vi "SIRRectHole.vi"(8 "P":cluster{"x":dbl, "y":dbl, "z":dbl}={"x"=1.0, "y"=-5.0, "z"=1.0} {"x" format="%.2f"; "z" format="%.2f"; "y" format="%.2f"}, 9 "Variables":T1={"sound spd (cm/s)"=150000, "time step (s)"=1e-09} {"time step (s)" format="%.2e"}, 11 "strip":cluster{"Radius":dbl, "h":dbl, "a":dbl}={"Radius"=10.0, "h"=3.0, "a"=5.0} {"Radius" format="%.2f"; "a" format="%.2f"; "h" format="%.2f"}) -> (1 "lower":dbl[](graph), 2 "upper":dbl[](graph), 3 "h rect":dbl[](graph), 4 "delay out":i32, 5 "h cap":dbl[](array[numeric]) format="%.2f", 7 "cap delay pts":i32)   [LabVIEW 2022 SP3]
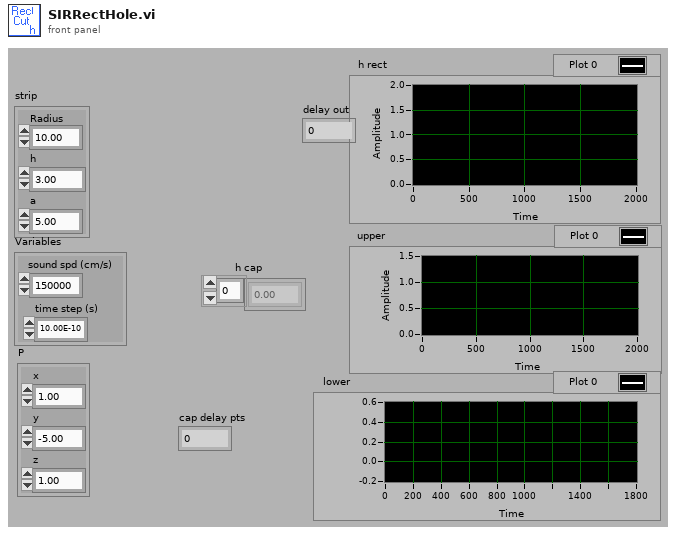
[diagram p1: front panel]
types:
  T1 = cluster{"sound spd (cm/s)":i32, "time step (s)":sgl}
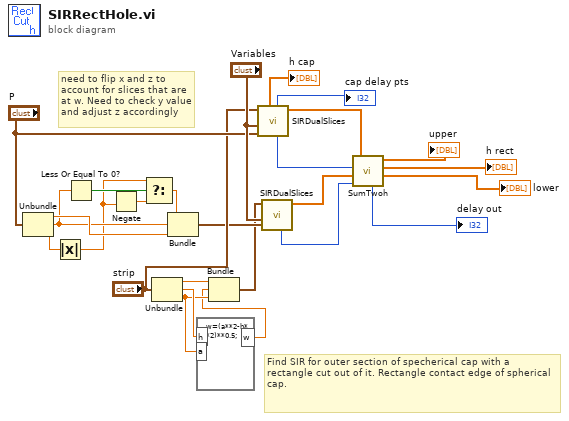
[diagram p0: block diagram]
diagram:
  # "need to flip x and z to account for slices that are at w. Need to check y value and adjust z accordingly"
  # "Find SIR for outer section of specherical cap with a rectangle cut out of it. Rectangle contact edge of spherical cap."
  n1 = Unbundle("P") -> ("x"=w13:dbl, "y"=w5:dbl, "z"=w12:dbl)
  n2 = Absolute Value(x=w12) -> (abs(x)=w2:dbl)
  n3 = Less Or Equal To 0?(x=w5) -> (x <= 0?=w4:bool)
  n4 = Negate(x=w2) -> (-x=w3:dbl)
  n5 = Select(t=w2, s=w4, f=w3) -> (s? t:f=w1:dbl)
  n6 = Unbundle("strip") -> ("Radius"=w18:dbl, "h"=w17:dbl, "a"=w16:dbl)
  n7 = Bundle(w1, "y"=w5, "x"=w13) -> (w11:cluster{dbl, "y":dbl, "x":dbl})  [unwired: 1 out]
  n8 = formula code="w=(a**2-h**2)**0.5;"("h"=w17, "a"=w16) -> ("w"=w14:dbl)
  n9 = Bundle("Radius"=w18, "w"=w14, "a"=w16) -> (w10:cluster{"Radius":dbl, "w":dbl, "a":dbl})  [unwired: 1 out]
  n10 = call "SIRDualSlices.vi"("P"="P", "Variables"="Variables", "strip"="strip") -> ("h outer strips"=w25:dbl[], "delay out"=w23:i32, "cap delay pts"=→"cap delay pts":i32, "h cap"=→"h cap":dbl[])  [unwired: 5 out]
  n11 = call "SIRDualSlices.vi"("P"=w11, "Variables"="Variables", "strip"=w10) -> ("h outer strips"=w24:dbl[], "delay out"=w22:i32)  [unwired: 7 out]
  n12 = call "SumTwoh.vi"("h1"=w25, "delay1"=w23, "h2"=w24, "delay2"=w22) -> ("delay out"=→"delay out":i32, "upper"=→"upper":dbl[], "h sum"=→"h rect":dbl[], "lower"=→"lower":dbl[])  [unwired: 1 out]
